vi "str array to text).vi"(11 "Array":string[](array[string])=["laythw", "_-view o t", "-plot y ", "PublishToWeb PNG.pc3", "VGA (480.00 x 640.00 Pixels)", "l n e F", " .", "y  D:\\inetpub\\wwwroot\\Designs\\LFOM\\5116\\50Lps\\LFOMTemplate", "n y", "shademode x -view swiso", ""]) -> (3 "String":string)   [LabVIEW 2012, in "Design Server.lvlib"]
uses:
  Design Server.lvlib
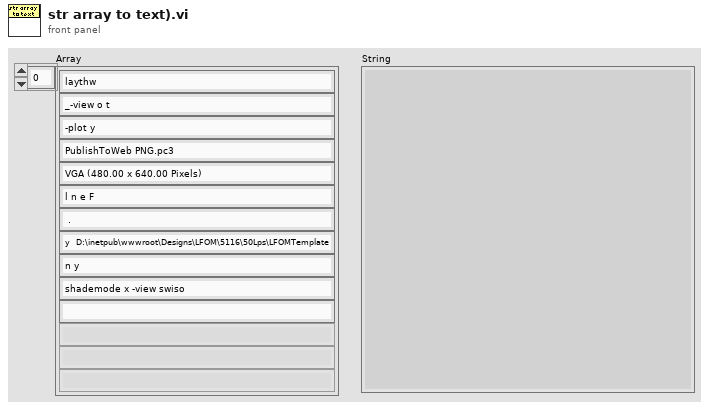
[diagram p1: front panel]
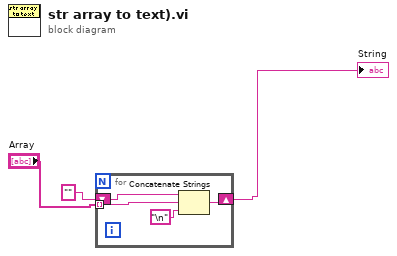
[diagram p0: block diagram]
diagram:
  n1 = for {
    tunnel: "Array" -> [w5] mode=indexing
    shift-right: [w6] -> w3
    shift-left: "" -> [w7]
    n2 = Concatenate Strings(w7, w5, "\n") -> (w6:string)
  }
  "String" <- w3
